vi "Rotation2d_UnaryMinus.vi"(11 "in ROTATION":T1 {"SIN" format="%13.4f"; "COS" format="%13.4f"; "VALUE" format="%13.4f"}) -> (3 "out ROTATION":T1 {"SIN" format="%13.4f"; "COS" format="%13.4f"; "VALUE" format="%13.4f"})   [LabVIEW 2019, in "Trajectory_Library.lvlib"]
doc: "Takes the inverse of the current rotation. This is simply the negative of the current angular value.\n\nParameters:\n - IN ROTATION - This ROTATION data structure\n\nResults:\n - OUT ROTATION - The negated ROTATION data structure."
uses:
  Trajectory_Library.lvlib
  TypeDef/ROTATION2D.ctl
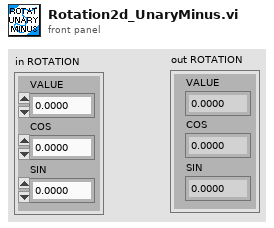
[diagram p1: front panel]
types:
  T1 = typedef "Trajectory_Library.lvlib/ROTATION2D.ctl" = cluster{"VALUE":dbl, "COS":dbl, "SIN":dbl}
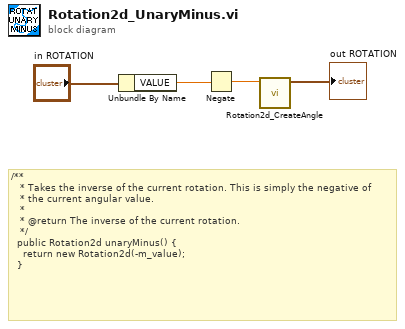
[diagram p0: block diagram]
diagram:
  # "/**\n   * Takes the inverse of the current rotation. This is simply the negative of\n   * the current angular value.\n   *\n   * @return The inverse of the current rotation.\n   */\n  public Rotation2d unaryMinus() {\n    return new Rotation2d(-m_value);\n  }"
  n1 = Unbundle By Name("in ROTATION") -> ("VALUE"=w3:dbl)
  n2 = Negate(x=w3) -> (-x=w2:dbl)
  n3 = call "Rotation2d_CreateAngle.vi"("Angle"=w2) -> ("ROTATION"=→"out ROTATION":T1)  [unwired: 10 in]
